vi "LEBITplc.SendError.vi"(0 "i ref in":refnum<vi>, 2 "Index":i32[](array[numeric]), 5 "error IO":errorcluster) -> (14 "i ref out":refnum<vi>, 19 "error out":errorcluster)   [LabVIEW 2012, in "LEBITplc.lvlib"]
uses:
  LEBITplc.lvlib
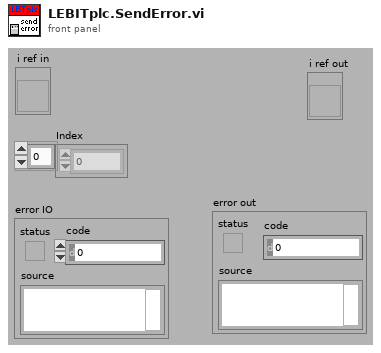
[diagram p1: front panel]
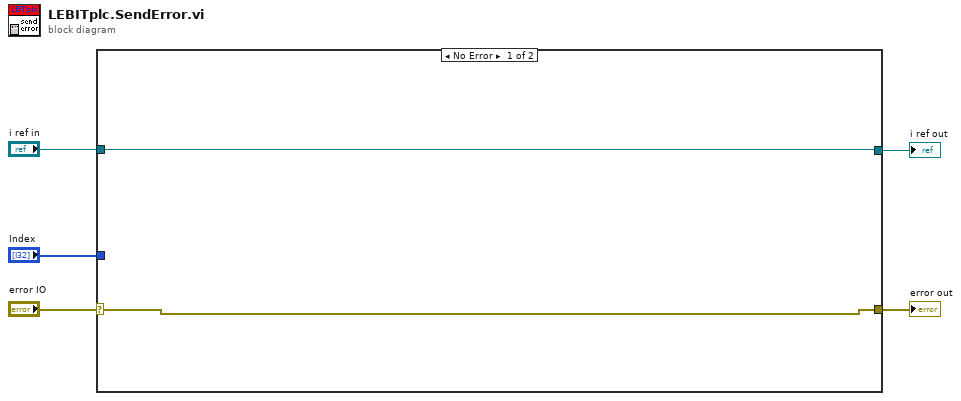
[diagram p0: block diagram]
diagram:
  n1 = case shown="No Error" "error IO" {
    selector: "error IO" -> [w6 w8]
    tunnel: "i ref in" -> [w7 w9]
    tunnel: [w6 w8] -> w4
    tunnel: [w7 w9] -> w3
    tunnel: "Index" -> [_ _]
    frame No Error {
    }
    frame Error {
    }
  }
  "error out" <- w4
  "i ref out" <- w3
